vi "Send command Set Pin.vi"(0 "Simulado in":refnum<class "Simulado.lvclass">, 1 "Puerto":string(combo), 2 "Pin":string(combo), 3 "Valor":string(combo), 5 "error in (no error)":errorcluster, 6 "Marca":string) -> (14 "Simulado out":refnum<class "Simulado.lvclass">, 16 "Command":string, 17 "Expected response":string, 19 "error out":errorcluster)   [LabVIEW 2020, in "Simulado.lvclass"]
uses:
  Simulado.lvclass
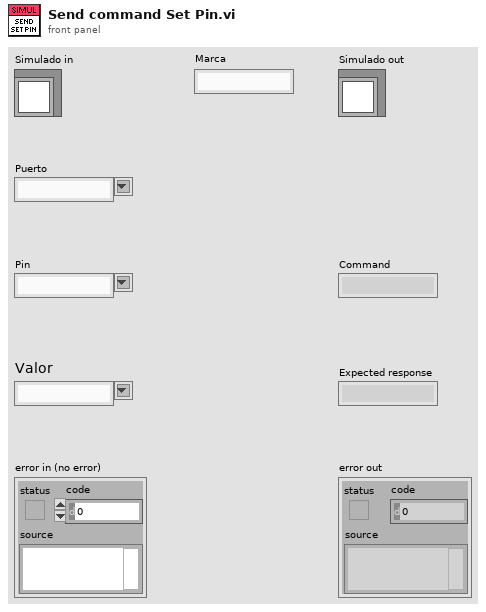
[diagram p1: front panel]
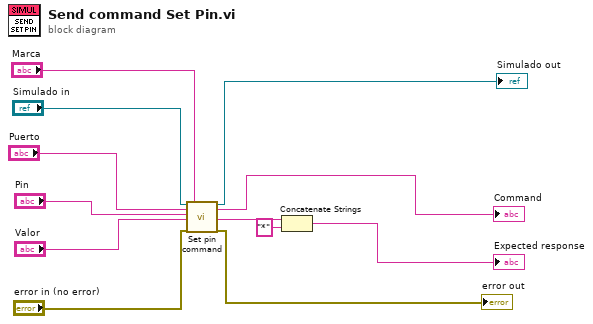
[diagram p0: block diagram]
diagram:
  n1 = call-dynamic "Set pin command.vi"("Serial Device in"="Simulado in", "Puerto"="Puerto", "Pin"="Pin", "Valor"="Valor", "error in (no error)"="error in (no error)", "Marca"="Marca") -> ("Serial Device out"=→"Simulado out":refnum<class "Simulado.lvclass">, "Command"=→"Command":string, "Expected response"=w3:string, "error out"=→"error out":errorcluster)  [unwired: 10 in]
  n2 = Concatenate Strings(w3, "*" ("string")) -> (→"Expected response":string)
